vi "Initialize.vi"(7 "Serial Configuration":T1={"Baud Rate"=57600, "Parity"=1, "Data Bits"=7, "Stop Bits"=10, "Flow Control"=0} {"Flow Control" items=["None", "XON/XOFF", "RTS/CTS", "XON/XOFF & RTS/CTS", "DTR/DSR", "XON/XOFF & DTR/DSR"]; "Stop Bits" items=["1.0"=10, "1.5"=15, "2.0"=20]; "Data Bits" items=["7"=7, "8"=8]; "Parity" items=["None", "Odd", "Even", "Mark", "Space"]; "Baud Rate" items=["300"=300, "600"=600, "1200"=1200, "2400"=2400, "4800"=4800, "9600"=9600, "19200"=19200, "38400"=38400, "57600"=57600]}, 8 "error in (no error)":errorcluster, 9 "Reset (True)":bool=TRUE, 10 "ID Query (True)":bool=TRUE, 11 "VISA resource name":refnum<visa-resource-name>) -> (0 "error out":errorcluster, 3 "VISA resource name out":refnum<visa-resource-name>)   [LabVIEW 2019, in "Lake Shore 335.lvlib"]
doc: "Establishes communication with the instrument and optionally performs an instrument identification query and/or an instrument reset. It also places the instrument in a default state needed for other instrument driver operations. Therefore, call this VI before calling other instrument driver VIs for this instrument. Generally, you need to call the <B>Initialize VI</B> only once at the beginning of an application."
uses:
  <instrlib>/Lake Shore 335/Lake Shore 335.lvlib
panel:
  # "(c) 2011 Lake Shore Cryotronics Inc.  ALL RIGHTS RESERVED."
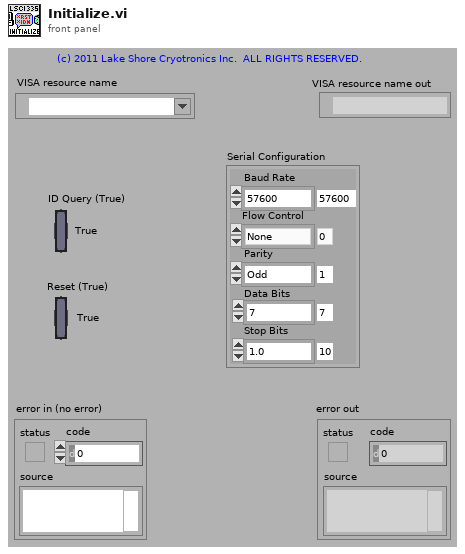
[diagram p1: front panel]
types:
  T1 = cluster{"Baud Rate":u32, "Parity":u16, "Data Bits":u16, "Stop Bits":u16, "Flow Control":u16}
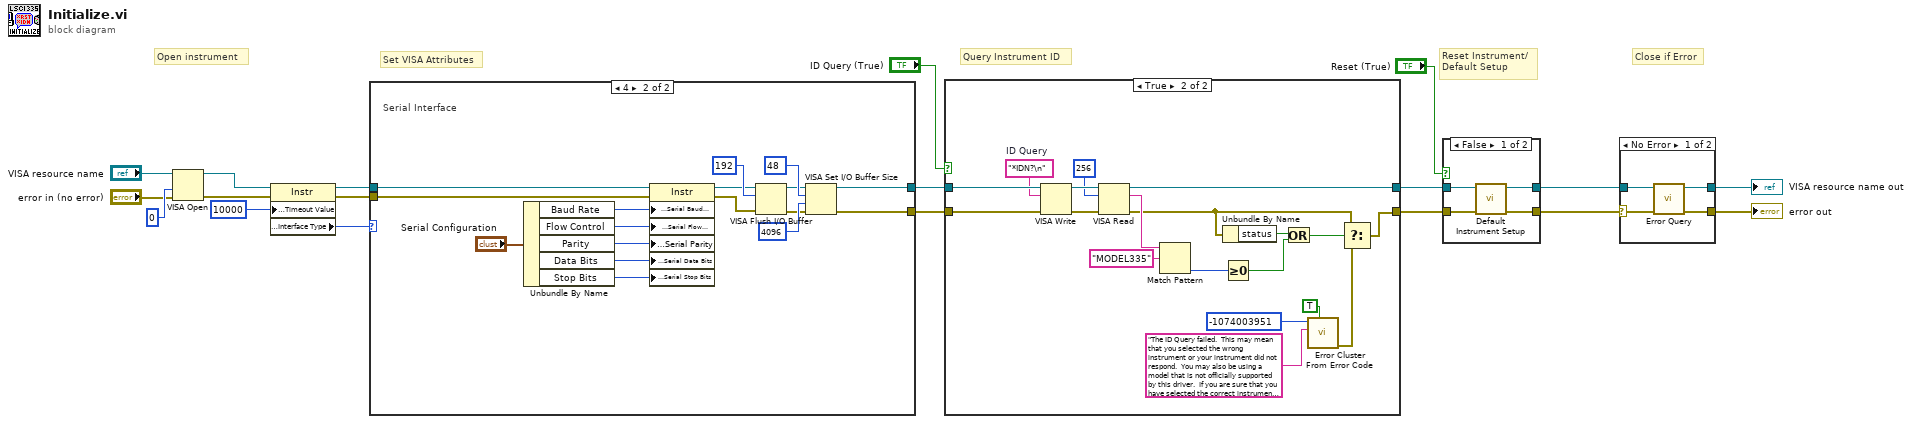
[diagram p0: block diagram]
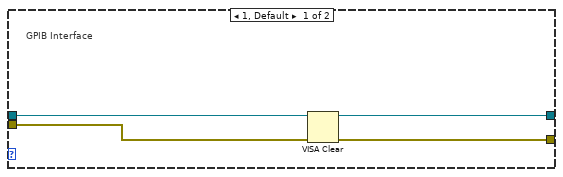
[diagram p2: hidden frame]
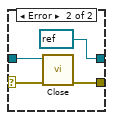
[diagram p3: hidden frame]
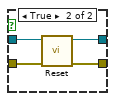
[diagram p4: hidden frame]
diagram:
  # "Set VISA Attributes"
  # "Close if Error"
  # "Query Instrument ID"
  # "Reset Instrument/\nDefault Setup"
  # "Open instrument"
  n1 = VISA Open(access mode=u32 0, error in (no error)="error in (no error)", VISA resource name="VISA resource name") -> (VISA resource name=w9:refnum<visa-resource-name>, error out=w8:errorcluster)  [unwired: 2 in]
  n2 = property class="Instr"(reference=w9, error in=w8, "General Settings:Timeout Value"=u32 10000) -> (reference out=w7:refnum<visa-resource-name>, error out=w6:errorcluster, "Interface Information:Interface Type"=w5:u16)
  n3 = case shown="4" w5 {
    tunnel: [w23 w27] -> w2
    tunnel: [w22 w26] -> w1
    tunnel: w7 -> [w20 w24]
    tunnel: w6 -> [w21 w25]
    frame 1, Default {
      # "GPIB Interface"
      n4 = VISA Clear(VISA resource name=w20, error in (no error)=w21) -> (VISA resource name out=w23:refnum<visa-resource-name>, error out=w22:errorcluster)
    }
    frame 4 {
      # "Serial Interface"
      n5 = Unbundle By Name("Serial Configuration") -> ("Baud Rate"=w35:u32, "Flow Control"=w39:u16, "Parity"=w37:u16, "Data Bits"=w36:u16, "Stop Bits"=w40:u16)
      n6 = property class="Instr"(reference=w24, error in=w25, "Serial Settings:Serial Baud Rate"=w35, "Serial Settings:Serial Flow Control"=w39, "Serial Settings:Serial Parity"=w37, "Serial Settings:Serial Data Bits"=w36, "Serial Settings:Serial Stop Bits"=w40) -> (reference out=w31:refnum<visa-resource-name>, error out=w29:errorcluster)
      n7 = VISA Flush I/O Buffer(VISA resource name=w31, mask (16)=u16 192, error in (no error)=w29) -> (VISA resource name out=w28:refnum<visa-resource-name>, error out=w30:errorcluster)
      n8 = VISA Set I/O Buffer Size(VISA resource name=w28, mask (16)=u16 48, size (4096)=u32 4096 ("size (0)"), error in (no error)=w30) -> (VISA resource name out=w27:refnum<visa-resource-name>, error out=w26:errorcluster)
    }
  }
  n9 = case shown="True" "ID Query (True)" {
    tunnel: [w41 w61] -> w18
    tunnel: [w42 w44] -> w19
    tunnel: w2 -> [w42 w59]
    tunnel: w1 -> [w41 w60]
    frame False {
    }
    frame True {
      w45 = "*IDN?\n"  # ID Query
      n10 = VISA Write(VISA resource name=w59, write buffer=w45, error in (no error)=w60) -> (VISA resource name out=w57:refnum<visa-resource-name>, error out=w56:errorcluster)  [unwired: 1 out]
      n11 = VISA Read(VISA resource name=w57, byte count=u32 256, error in (no error)=w56) -> (VISA resource name out=w44:refnum<visa-resource-name>, read buffer=w58:string, error out=w43:errorcluster)  [unwired: 1 out]
      n12 = Match Pattern(string=w58, regular expression="MODEL335") -> (offset past match=w49:i32)  [unwired: 1 in, 3 out]
      n13 = Unbundle By Name(w43) -> ("status"=w48:bool)
      n14 = Greater Or Equal To 0?(x=w49) -> (x >= 0?=w46:bool)
      n15 = Or(x=w48, y=w46) -> (x .or. y?=w47:bool)
      n16 = call <vilib>:"Error Cluster From Error Code.vi"("show call chain? (False)"=TRUE, "error message (\"\")"="The ID Query failed.  This may mean that you selected the wrong instrument or your instrument did not respond.  You may also be using a model that is not officially supported by this driver.  If you are sure that you have selected the correct instrument and it is responding, try disabling the ID Query." ("Source (VI Name)"), "error code (0)"=-1074003951 ("Code")) -> ("error out"=w53:errorcluster)  [unwired: 6 in]
      n17 = Select(t=w43, s=w47, f=w53) -> (s? t:f=w61:errorcluster)
    }
  }
  n18 = case shown="False" "Reset (True)" {
    tunnel: w18 -> [w64 w66]
    tunnel: [w63 w69] -> w12
    tunnel: w19 -> [w65 w67]
    tunnel: [w62 w68] -> w13
    frame False {
      n19 = call <instrlib>:"Default Instrument Setup.vi"("error in (no error)"=w64, "VISA resource name"=w65) -> ("error out"=w63:errorcluster, "VISA resource name out"=w62:refnum<visa-resource-name>)  [unwired: 8 in]
    }
    frame True {
      n20 = call <instrlib>:"Reset.vi"("error in (no error)"=w66, "VISA resource name"=w67) -> ("error out"=w69:errorcluster, "VISA resource name out"=w68:refnum<visa-resource-name>)  [unwired: 8 in]
    }
  }
  n21 = case shown="No Error" w12 {
    selector: w12 -> [w73 w75]
    tunnel: w13 -> [w72 w76]
    tunnel: [w71 refnum<visa-resource-name> refnum ("VISA resource name out")] -> w15
    tunnel: [w70 w77] -> w14
    frame No Error {
      n22 = call <instrlib>:"Error Query.vi"("error in (no error)"=w73, "VISA resource name"=w72) -> ("error out"=w70:errorcluster, "VISA resource name out"=w71:refnum<visa-resource-name>)  [unwired: 7 in, 1 out]
    }
    frame Error {
      n23 = call <instrlib>:"Close.vi"("error in (no error)"=w75, "VISA resource name"=w76) -> ("error out"=w77:errorcluster)  [unwired: 9 in]
    }
  }
  "VISA resource name out" <- w15
  "error out" <- w14
